vi "Test save Scande.vi"() -> ()   [LabVIEW 2020]
uses:
  Labview Library/Libraries/Basic Experiment/Scan Settings.ctl
  Axis Enum.ctl
  Labview Library/Libraries/Basic Experiment/Basic Experiment.lvlib
  Labview Library/Libraries/LaoJi/UT_Utilities/Utilities.lvlib
panel:
  in  "file path":path=path "G:/Default/Save/demo Save_Y2021_M12_D01_21_20_53.tdms"
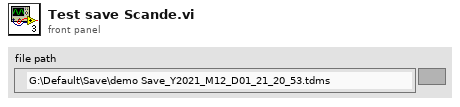
[diagram p1: front panel]
types:
  T1 = typedef "Basic Experiment.lvlib/Scan Settings.ctl" = cluster{"Horizontal axis":T2, "Vertical axis":T2, "vertical num":u32, "vertical end":dbl, "vertical start":dbl, "horizontal num":u32, "horizontal end":dbl, "horizontal start":dbl}
  T2 = typedef "Axis Enum.ctl" = enum16{"x", "y", "z"}
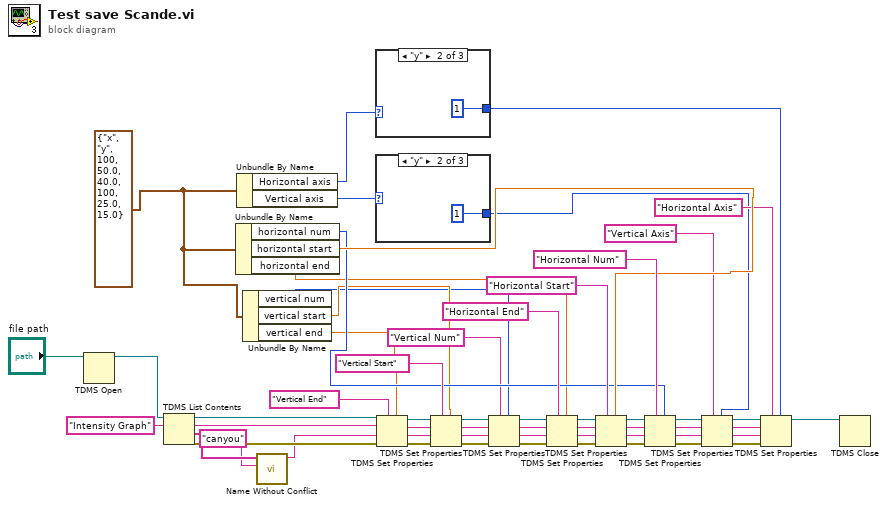
[diagram p0: block diagram]
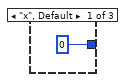
[diagram p2: hidden frame]
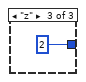
[diagram p3: hidden frame]
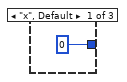
[diagram p4: hidden frame]
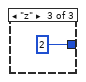
[diagram p5: hidden frame]
diagram:
  w4 = T1 {"Horizontal axis"=enum."x", "Vertical axis"=enum."y", "vertical num"=100, "vertical end"=50.0, "vertical start"=40.0, "horizontal num"=100, "horizontal end"=25.0, "horizontal start"=15.0} ("Scan parameter")
  n1 = TDMS Open(11:"file path") -> (3:w9:refnum<k34>)  [unwired: 6 in, 1 out]
  n2 = TDMS List Contents(6:"Intensity Graph" ("group name"), 7:w9) -> (0:w6:errorcluster, 1:w3:string[], 2:w11:string, 3:w5:refnum<k34>)  [unwired: 1 in]
  n3 = Unbundle By Name(w4) -> ("horizontal num"=w36:u32, "horizontal start"=w37:dbl, "horizontal end"=w15:dbl)
  n4 = Unbundle By Name(w4) -> ("Horizontal axis"=w19:T2, "Vertical axis"=w18:T2)
  n5 = Unbundle By Name(w4) -> ("vertical num"=w12:u32, "vertical start"=w14:dbl, "vertical end"=w13:dbl)
  n6 = call "Name Without Conflict.vi"("name"="canyou", "Exist Name Array"=w3) -> ("New Name"=w2:string)  [unwired: 9 in]
  n7 = case shown="\"y\"" w19 {
    tunnel: [0 1 2] -> w17
    frame "x", Default {
    }
    frame "y" {
    }
    frame "z" {
    }
  }
  n8 = case shown="\"y\"" w18 {
    tunnel: [0 1 2] -> w16
    frame "x", Default {
    }
    frame "y" {
    }
    frame "z" {
    }
  }
  n9 = TDMS Set Properties(5:w13, 7:"Vertical End" ("group name in (Untitled)"), 8:w6, 9:w2, 10:w11, 11:w5) -> (0:w57:errorcluster, 1:w56:string, 2:w55:string, 3:w54:refnum<k34>)
  n10 = TDMS Set Properties(5:w14, 7:"Vertical Start" ("group name in (Untitled)"), 8:w57, 9:w56, 10:w55, 11:w54) -> (0:w52:errorcluster, 1:w51:string, 2:w50:string, 3:w49:refnum<k34>)
  n11 = TDMS Set Properties(5:w12, 7:"Vertical Num" ("group name in (Untitled)"), 8:w52, 9:w51, 10:w50, 11:w49) -> (0:w41:errorcluster, 1:w42:string, 2:w43:string, 3:w44:refnum<k34>)
  n12 = TDMS Set Properties(5:w15, 7:"Horizontal End" ("group name in (Untitled)"), 8:w41, 9:w42, 10:w43, 11:w44) -> (0:w45:errorcluster, 1:w46:string, 2:w21:string, 3:w22:refnum<k34>)
  n13 = TDMS Set Properties(5:w37, 7:"Horizontal Start" ("group name in (Untitled)"), 8:w45, 9:w46, 10:w21, 11:w22) -> (0:w47:errorcluster, 1:w48:string, 2:w20:string, 3:w23:refnum<k34>)
  n14 = TDMS Set Properties(5:w36, 7:"Horizontal Num" ("group name in (Untitled)"), 8:w47, 9:w48, 10:w20, 11:w23) -> (0:w33:errorcluster, 1:w32:string, 2:w31:string, 3:w30:refnum<k34>)
  n15 = TDMS Set Properties(5:w16, 7:"Vertical Axis" ("group name in (Untitled)"), 8:w33, 9:w32, 10:w31, 11:w30) -> (0:w29:errorcluster, 1:w28:string, 2:w27:string, 3:w26:refnum<k34>)
  n16 = TDMS Set Properties(5:w17, 7:"Horizontal Axis" ("group name in (Untitled)"), 8:w29, 9:w28, 10:w27, 11:w26) -> (3:w7:refnum<k34>)  [unwired: 3 out]
  n17 = TDMS Close(11:w7) -> ()  [unwired: 1 in, 2 out]
